vi "Create.vi"(10 "Config Info":T1) -> (3 "ConfigInfoValue out":refnum<class "ConfigInfoValue.lvclass">)   [LabVIEW 2020, in "Volatus.lvlib" / "ConfigInfoValue.lvclass"]
uses:
  ConfigInfoValue.lvclass
  ConfigInfoValue.lvclass/ConfigInfoValue.ctl
  Config Info.ctl
  Volatus.lvlib
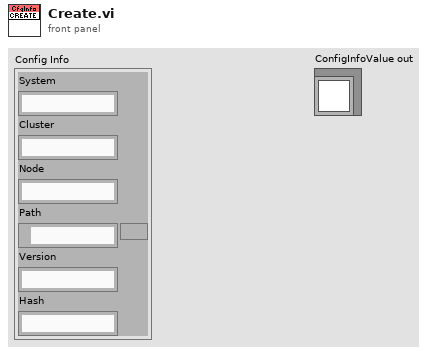
[diagram p1: front panel]
types:
  T1 = typedef "Volatus.lvlib/Config Info.ctl" = cluster{"System":string, "Cluster":string, "Node":string, "Path":path, "Version":string, "Hash":string}
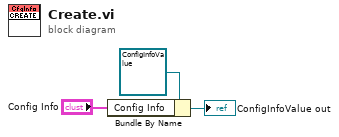
[diagram p0: block diagram]
diagram:
  n1 = Bundle By Name(cluster=refnum<class "ConfigInfoValue.lvclass"> refnum ("ConfigInfoValue in"), "Config Info"="Config Info") -> (→"ConfigInfoValue out":refnum<class "ConfigInfoValue.lvclass">)
